vi "installer_create_file_path.vi"(6 "build_spec_name":string, 8 "error in (no error)":errorcluster, 11 "distribution_folder":path) -> (0 "error out":errorcluster, 3 "path":path)   [LabVIEW 2015, in "lv-builder-default.lvlib"]
uses:
  lv-builder-default.lvlib
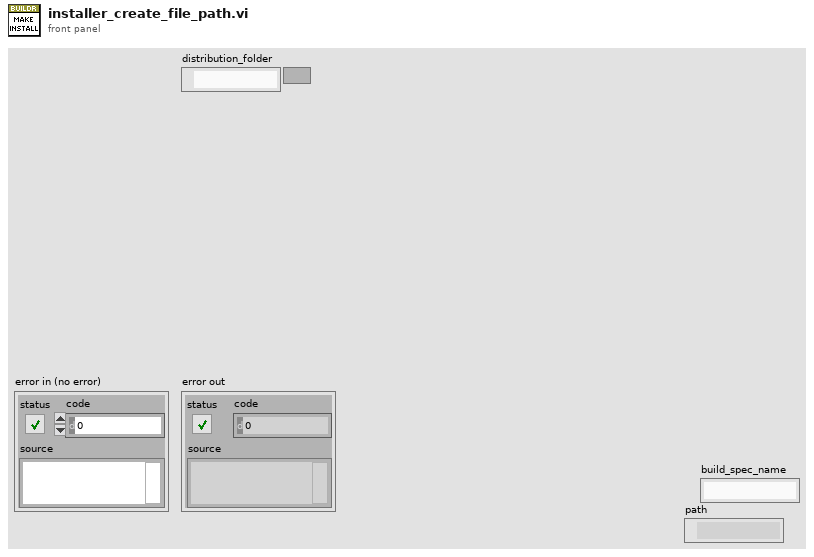
[diagram p1: front panel]
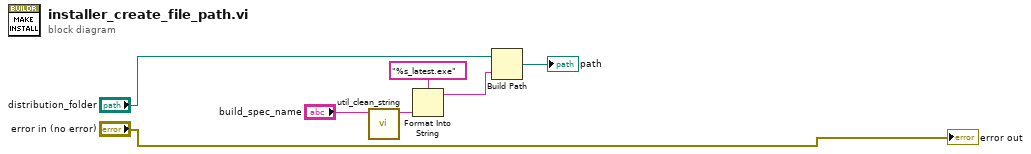
[diagram p0: block diagram]
diagram:
  n1 = call "util_clean_string.vi"("string"="build_spec_name") -> ("string_clean"=w3:string)  [unwired: 10 in]
  n2 = Format Into String(format string="%s_latest.exe", w3) -> (resulting string=w6:string)  [unwired: 2 in, 1 out]
  n3 = Build Path(base path="distribution_folder", name or relative path=w6) -> (appended path=→"path":path)
  "error out" <- "error in (no error)"
